vi "S7COMM - Build Data Array.vi"(10 "Data":u32[](array[numeric]), 11 "Variable Type":T3=enum."BIT") -> (2 "S7 Data (Byte Array)":T1 format="0x%02x", 3 "Data Length":u16)   [LabVIEW 2014, in "S7NetCom.lvclass"]
doc: "____\nCopyright (c) 2019 Hampel Software Engineering (HSE), released under BSD license. More info can be found on https://dokuwiki.hampel-soft.com/code/hse/s7netcom. Original code published by Marc Christenson, Sisu Devices."
uses:
  S7NetCom.lvclass
  Controls/S7_Variable_Type.ctl
  Controls/S7NetCom_HexByteArray.ctl
  Controls/S7NetCom_HexByte.ctl
  S7COMM - Transport Data Types--ring.ctl
panel:
  # "More info on https://dokuwiki.hampel-soft.com/code/hse/s7netcom\n\nCopyright (c) 2019, HAMPEL SOFTWARE ENGINEERING (HSE)\nOriginal code developed by Marc Christenson, Sisu Devices\nAll rights reserved.\n\nRedistribution and use in source and binary forms, with or without\nmodification, are permitted provided that the following conditions are met:\n\n1. Redistributions of source code must retain the above copyright\n   notice, this list of conditions and the following disclaimer.\n\n2. Redistributions in binary form must reproduce the above copyright\n   notice, this list of conditions and the following disclaimer in the\n   documentation and/or other materials provided with the distribution.\n\n3. All advertising materials mentioning features or use of this software\n   must display the following acknowledgement:\n   This product includes software developed by HAMPEL SOFTWARE ENGINEERING.\n\n4. Neither the name of HAMPEL SOFTWARE ENGINEERING nor the\n   names of its contributors may be used to endorse or promote products\n   derived from this software without specific prior written permission.\n\nTHIS SOFTWARE IS PROVIDED BY HAMPEL SOFTWARE ENGINEERING ''AS IS'' AND ANY\nEXPRESS OR IMPLIED WARRANTIES, INCLUDING, BUT NOT LIMITED TO, THE IMPLIED\nWARRANTIES OF MERCHANTABILITY AND FITNESS FOR A PARTICULAR PURPOSE ARE\nDISCLAIMED. IN NO EVENT SHALL HAMPEL SOFTWARE ENGINEERING BE LIABLE FOR ANY\nDIRECT, INDIRECT, INCIDENTAL, SPECIAL, EXEMPLARY, OR CONSEQUENTIAL DAMAGES\n(INCLUDING, BUT NOT LIMITED TO, PROCUREMENT OF SUBSTITUTE GOODS OR SERVICES;\nLOSS OF USE, DATA, OR PROFITS; OR BUSINESS INTERRUPTION) HOWEVER CAUSED AND\nON ANY THEORY OF LIABILITY, WHETHER IN CONTRACT, STRICT LIABILITY, OR TORT\n(INCLUDING NEGLIGENCE OR OTHERWISE) ARISING IN ANY WAY OUT OF THE USE OF THIS\nSOFTWARE, EVEN IF ADVISED OF THE POSSIBILITY OF SUCH DAMAGE."
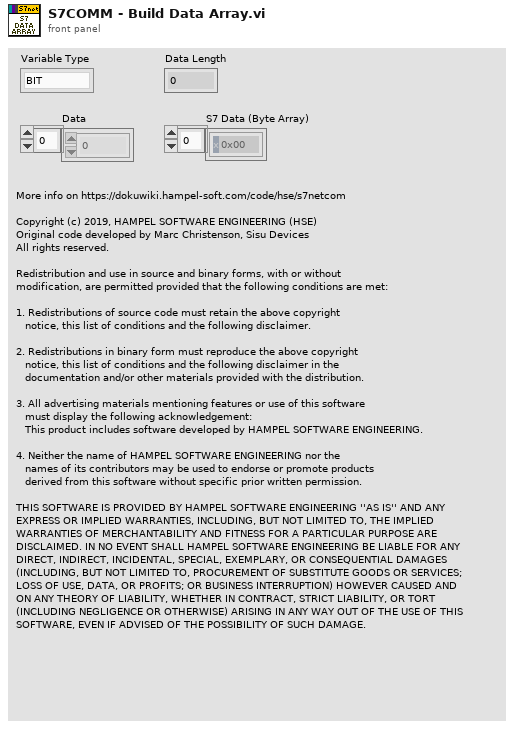
[diagram p1: front panel]
types:
  T1 = typedef "S7NetCom.lvclass/S7NetCom_HexByteArray.ctl" = T2[]
  T2 = typedef "S7NetCom.lvclass/S7NetCom_HexByte.ctl" = u8
  T3 = typedef "S7NetCom.lvclass/S7_Variable_Type.ctl" = enum8{"---", "BIT", "BYTE", "CHAR", "WORD", "INT", "DWORD", "DINT", "REAL"}
  T4 = typedef "S7NetCom.lvclass/S7COMM - Transport Data Types--ring.ctl" = u8
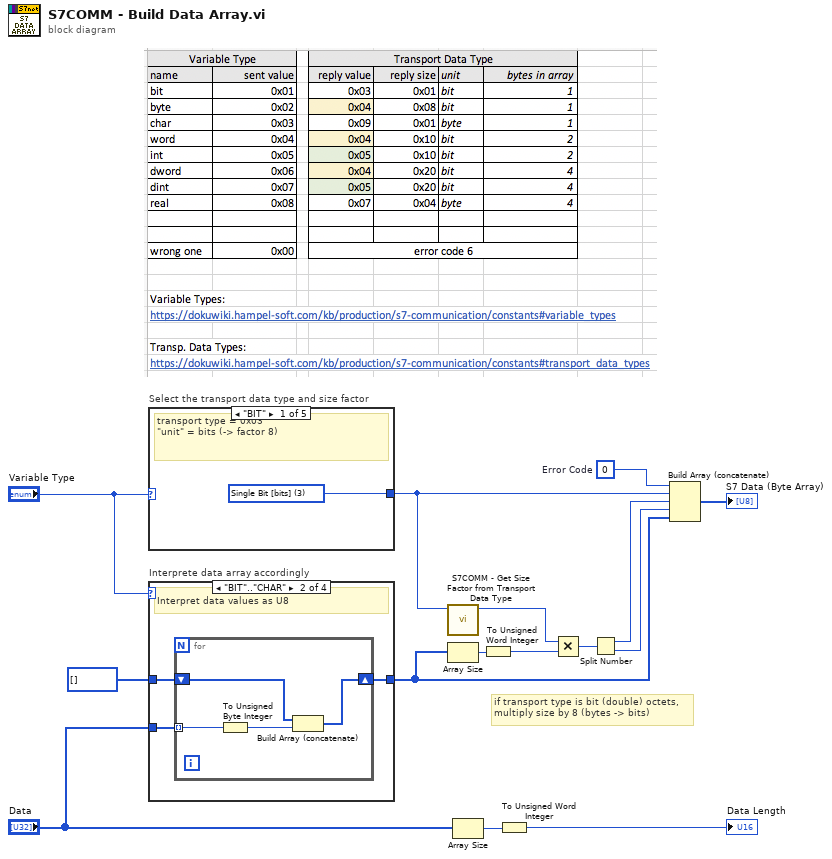
[diagram p0: block diagram]
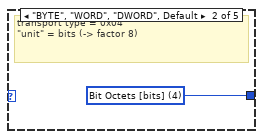
[diagram p2: hidden frame]
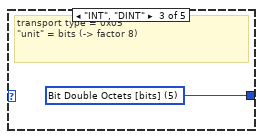
[diagram p3: hidden frame]
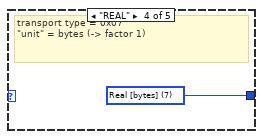
[diagram p4: hidden frame]
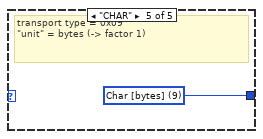
[diagram p5: hidden frame]
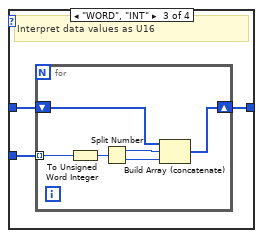
[diagram p7: hidden frame]
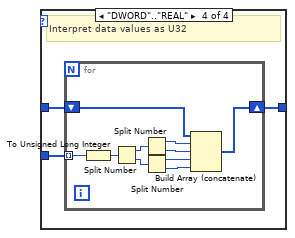
[diagram p8: hidden frame]
diagram:
  w4 = T2 0  # Error Code
  # "if transport type is bit (double) octets,\nmultiply size by 8 (bytes -> bits)"
  n1 = case "Select the transport data type and size factor" shown="\"BIT\"" "Variable Type" {
    tunnel: [w16 w17 w18 w19 w20] -> w2
    frame "BIT" {
      w16 = T4 3 items=["Single Bit [bits]"=3, "Bit Octets [bits]"=4, "Bit Double Octets [bits]"=5, "Real [bytes]"=7, "Char [bytes]"=9] ("Reply Data Types")
      # "transport type = 0x03\n\"unit\" = bits (-> factor 8)"
    }
    frame "BYTE", "WORD", "DWORD", Default {
      w17 = T4 4 items=["Single Bit [bits]"=3, "Bit Octets [bits]"=4, "Bit Double Octets [bits]"=5, "Real [bytes]"=7, "Char [bytes]"=9] ("Reply Data Types")
      # "transport type = 0x04\n\"unit\" = bits (-> factor 8)"
    }
    frame "INT", "DINT" {
      w18 = T4 5 items=["Single Bit [bits]"=3, "Bit Octets [bits]"=4, "Bit Double Octets [bits]"=5, "Real [bytes]"=7, "Char [bytes]"=9] ("Reply Data Types")
      # "transport type = 0x05\n\"unit\" = bits (-> factor 8)"
    }
    frame "REAL" {
      w19 = T4 7 items=["Single Bit [bits]"=3, "Bit Octets [bits]"=4, "Bit Double Octets [bits]"=5, "Real [bytes]"=7, "Char [bytes]"=9] ("Reply Data Types")
      # "transport type = 0x07\n\"unit\" = bytes (-> factor 1)"
    }
    frame "CHAR" {
      w20 = T4 9 items=["Single Bit [bits]"=3, "Bit Octets [bits]"=4, "Bit Double Octets [bits]"=5, "Real [bytes]"=7, "Char [bytes]"=9] ("Reply Data Types")
      # "transport type = 0x09\n\"unit\" = bytes (-> factor 1)"
    }
  }
  n2 = case "Interprete data array accordingly" shown="\"BIT\"..\"CHAR\"" "Variable Type" {
    tunnel: [w21 w24 w31 w40] -> w10
    tunnel: "Data" -> [_ w22 w30 w39]
    tunnel: T1 [] ("Array") -> [w21 w23 w29 w38]
    frame Default {
    }
    frame "BIT".."CHAR" {
      # "Interpret data values as U8"
      n3 = for {
        shift-right: [w28] -> w24
        shift-left: w23 -> [w27]
        tunnel: w22 -> [w26] mode=indexing
        n4 = To Unsigned Byte Integer(number=w26) -> (unsigned 8bit integer=w25:u8)
        n5 = Build Array (concatenate)(w27, w25) -> (w28:T1)
      }
    }
    frame "WORD", "INT" {
      # "Interpret data values as U16"
      n6 = for {
        tunnel: w30 -> [w33] mode=indexing
        shift-right: [w37] -> w31
        shift-left: w29 -> [w32]
        n7 = To Unsigned Word Integer(number=w33) -> (unsigned 16bit integer=w34:u16)
        n8 = Split Number(x=w34) -> (hi(x)=w36:u8, lo(x)=w35:u8)
        n9 = Build Array (concatenate)(w32, w36, w35) -> (w37:T1)
      }
    }
    frame "DWORD".."REAL" {
      # "Interpret data values as U32"
      n10 = for {
        tunnel: w39 -> [w42] mode=indexing
        shift-right: [w50] -> w40
        shift-left: w38 -> [w41]
        n11 = To Unsigned Long Integer(number=w42) -> (unsigned 32bit integer=w43:u32)
        n12 = Split Number(x=w43) -> (hi(x)=w49:u16, lo(x)=w48:u16)
        n13 = Split Number(x=w49) -> (hi(x)=w47:u8, lo(x)=w46:u8)
        n14 = Split Number(x=w48) -> (hi(x)=w44:u8, lo(x)=w45:u8)
        n15 = Build Array (concatenate)(w41, w47, w46, w44, w45) -> (w50:T1)
      }
    }
  }
  n16 = call "S7COMM - Get Size Factor from Transport Data Type.vi"("Transport Data Type"=w2) -> ("Size Factor"=w1:u16)  [unwired: 10 in]
  n17 = Array Size(array=w10) -> (size(s)=w5:i32)
  n18 = Array Size(array="Data") -> (size(s)=w11:i32)
  n19 = To Unsigned Word Integer(number=w5) -> (unsigned 16bit integer=w9:u16)
  n20 = To Unsigned Word Integer(number=w11) -> (unsigned 16bit integer=→"Data Length":u16)
  n21 = Multiply(x=w1, y=w9) -> (x*y=w8:u16)
  n22 = Split Number(x=w8) -> (hi(x)=w6:u8, lo(x)=w7:u8)
  n23 = Build Array (concatenate)(w4, w2, w6, w7, w10) -> (→"S7 Data (Byte Array)":T1)
